vi "Get Splitter Size.vi"(8 "error in (no error)":errorcluster, 11 "Divider in":refnum<class "Divider.lvclass">) -> (0 "error out":errorcluster, 1 "Splitter size":i16, 2 ".5 Splitter size":i16, 3 "Divider out":refnum<class "Divider.lvclass">)   [LabVIEW 2013, in "Divider.lvclass"]
doc: "Copyright 2018, Wiebe Walstra, wiebe@carya.nl."
uses:
  Divider.lvclass
  Divider.lvclass/Divider.ctl
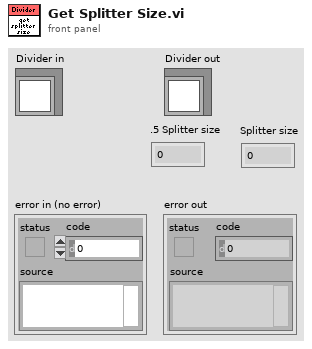
[diagram p1: front panel]
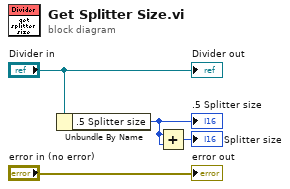
[diagram p0: block diagram]
diagram:
  n1 = Unbundle By Name("Divider in") -> (".5 Splitter size"=w1:i16)
  ".5 Splitter size" <- w1
  n2 = Add(x=w1, y=w1) -> (x+y=→"Splitter size":i16)
  "error out" <- "error in (no error)"
  "Divider out" <- "Divider in"
